vi "Set Enable State on Multiple Controls.vi"(8 "错误输入":cluster{"状态":bool, "代码":i32, "源":string}, 10 "已禁用状态":T1(ring), 11 "控件":refnum<vi>[](array[refnum])) -> (0 "错误输出":cluster{"状态":bool, "代码":i32, "源":string})   [LabVIEW 2012]
doc: "将输入数组中所有控件的值设置为“启用状态”。"
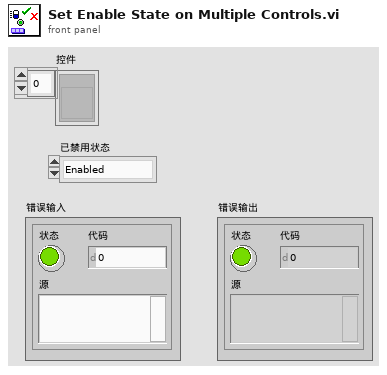
[diagram p1: front panel]
types:
  T1 = enum8{"Enabled", "Disabled", "Disabled and Grayed Out"}
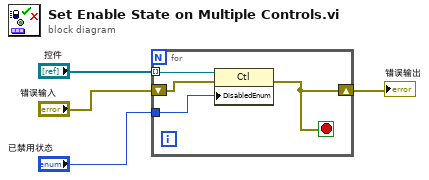
[diagram p0: block diagram]
diagram:
  n1 = for {
    tunnel: "控件" -> [w8] mode=indexing
    tunnel: "已禁用状态" -> [w7]
    shift-right: [w5] -> w3
    shift-left: "错误输入" -> [w6]
    stop <- w5 stop-if-true
    n2 = property on="属性节点" class="Ctl"(reference=w8, error in=w6, "DisabledEnum"=w7) -> (error out=w5:errorcluster)  [unwired: 1 out]
  }
  "错误输出" <- w3
